vi "Read PING))) Sensor Distance.vi"(8 "error in (no error)":errorcluster, 10 "default distance (NaN)":dbl=nan, 11 "starter kit host in":refnum<class "NI_Robotics_Starter Kit Host.lvclass">) -> (0 "error out":errorcluster, 1 "timed out?":bool, 2 "distance (m)":dbl, 3 "starter kit host out":refnum<class "NI_Robotics_Starter Kit Host.lvclass">)   [LabVIEW 2017, in "NI_Robotics_Starter Kit Host.lvclass"]
doc: "<B>Owning Palette:</B> Starter Kit 1.0 VIs, Starter Kit 2.0 VIs\n\nReads and returns the distance between the PING))) ultrasonic distance sensor and the nearest obstacle the sensor detects. The PING))) sensor has a maximum detection range of three meters."
uses:
  <vilib>/robotics/Starter Kit/Host Interface/NI_Robotics_Starter Kit Host.lvclass
  <vilib>/robotics/Starter Kit/Host Interface/NI_Robotics_Starter Kit Host.lvclass/NI_Robotics_Starter Kit Host.ctl
  <instrlib>/Parallax PING)))/HAIOL/Parallax PING))).lvclass
  <vilib>/robotics/Utilities/NI_Robotics Utilities.lvlib
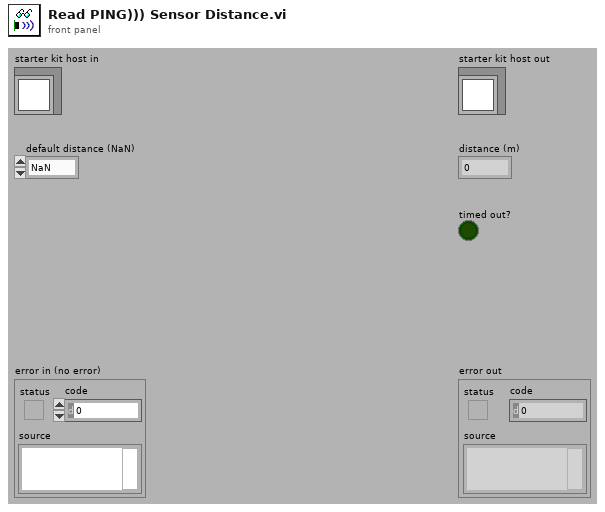
[diagram p1: front panel]
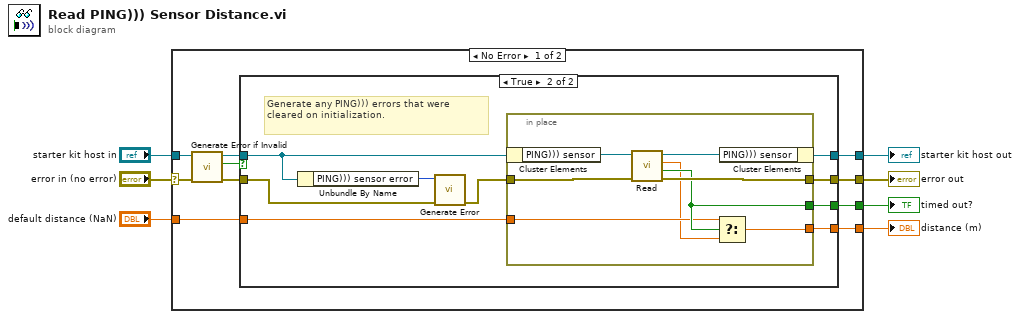
[diagram p0: block diagram]
diagram:
  n1 = case shown="No Error" "error in (no error)" {
    selector: "error in (no error)" -> [w10 w38]
    tunnel: [w14 w38] -> w6
    tunnel: [w17 w37] -> w4
    tunnel: "starter kit host in" -> [w12 w37]
    tunnel: [w16 _] -> w3
    tunnel: [w15 _] -> w2
    tunnel: "default distance (NaN)" -> [w13 _]
    frame No Error {
      n2 = call <vilib>:"Generate Error if Invalid.vi"("error in (no error)"=w10, "starter kit host in"=w12) -> ("error out"=w9:errorcluster, "valid?"=w8:bool, "starter kit host out"=w11:refnum<class "NI_Robotics_Starter Kit Host.lvclass">)  [unwired: 7 in]
      n3 = case shown="True" w8 {
        tunnel: [w19 w28] -> w17
        tunnel: [_ w27] -> w16
        tunnel: [_ w26] -> w15
        tunnel: [w18 w25] -> w14
        tunnel: w13 -> [_ w24]
        tunnel: w11 -> [w19 w23]
        tunnel: w9 -> [w18 w22]
        frame False {
        }
        frame True {
          # "Generate any PING))) errors that were cleared on initialization."
          n4 = Unbundle By Name(w23) -> ("PING))) sensor error"=w20:i32)
          n5 = call <vilib>:"Generate Error.vi"("error in (no error)"=w22, "code"=w20) -> ("error out"=w21:errorcluster)  [unwired: 9 in]
          n6 = in-place {
            in-place-border: [w29] -> w27
            in-place-border: [w32] -> w26
            in-place-border: w21 -> [w34]
            in-place-border: [w33] -> w25
            in-place-border: w24 -> [w31]
            n7 = in-place-cluster #1(w23) -> ("PING))) sensor"=w36:refnum<class "Parallax PING))).lvclass">)
            n8 = call-dynamic "Read.vi"("error in (no error)"=w34, "Parallax PING))) in"=w36) -> ("error out"=w33:errorcluster, "Timed out?"=w32:bool, "Distance (m)"=w30:dbl, "Parallax PING))) out"=w35:refnum<class "Parallax PING))).lvclass">)  [unwired: 6 in]
            n9 = Select(t=w31, s=w32, f=w30) -> (s? t:f=w29:dbl)
            n10 = in-place-cluster #1("PING))) sensor"=w35) -> (w28:refnum<class "NI_Robotics_Starter Kit Host.lvclass">)
          }
        }
      }
    }
    frame Error {
    }
  }
  "error out" <- w6
  "starter kit host out" <- w4
  "distance (m)" <- w3
  "timed out?" <- w2
